vi "add_cpath.vi"(8 "error in":errorcluster, 10 "string":string, 11 "lua_State *L":u64) -> (0 "error out":errorcluster)   [LabVIEW 2011]
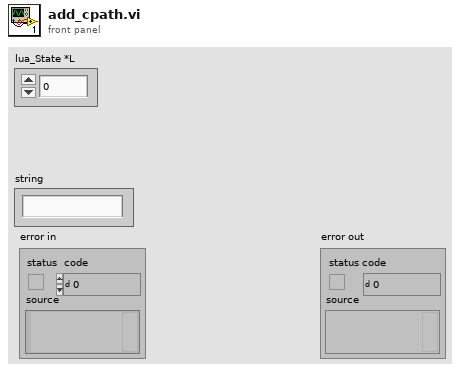
[diagram p1: front panel]
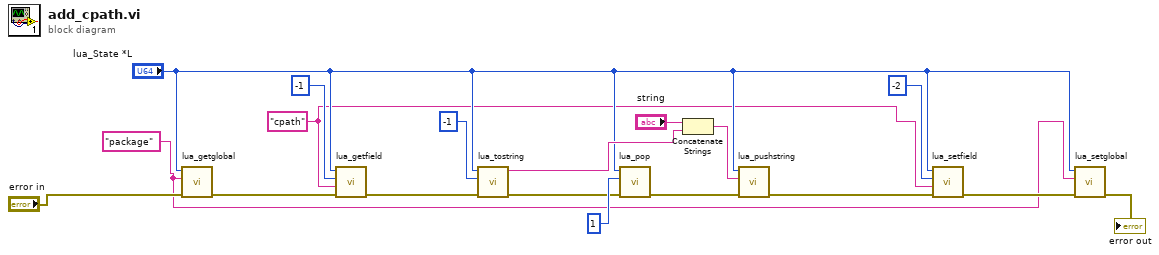
[diagram p0: block diagram]
diagram:
  w2 = "cpath" ("const char *name")
  w1 = "package" ("const char *name")
  n1 = call "lua_getglobal.vi"("error in"="error in", "const char *name"=w1, "lua_State *L"="lua_State *L") -> ("error out"=w9:errorcluster)  [unwired: 8 in]
  n2 = call "lua_getfield.vi"("error in"=w9, "const char *name"=w2, "int index"=-1, "lua_State *L"="lua_State *L") -> ("error out"=w11:errorcluster)  [unwired: 7 in]
  n3 = call "lua_tostring.vi"("error in"=w11, "index"=-1, "lua_State *L"="lua_State *L") -> ("error out"=w13:errorcluster, "constant string"=w12:string)  [unwired: 7 in]
  n4 = call "lua_pop.vi"("error in"=w13, "n"=1, "lua_State *L"="lua_State *L") -> ("error out"=w15:errorcluster)  [unwired: 8 in]
  n5 = Concatenate Strings("string", w12) -> (w16:string)
  n6 = call "lua_pushstring.vi"("error in"=w15, "const char *s"=w16, "lua_State *L"="lua_State *L") -> ("error out"=w18:errorcluster)  [unwired: 7 in, 1 out]
  n7 = call "lua_setfield.vi"("error in"=w18, "const char *k"=w2, "index"=-2, "lua_State *L"="lua_State *L") -> ("error out"=w6:errorcluster)  [unwired: 7 in]
  n8 = call "lua_setglobal.vi"("error in"=w6, "s"=w1, "lua_State *L"="lua_State *L") -> ("error out"=→"error out":errorcluster)  [unwired: 8 in]
